vi "qTSP.vi"(0 "System no.":i32=1 min=1 max=4 step=1, 2 "Sensor to query":string[](array[string]), 3 "All sensors?":bool, 4 "Sensor identifier?":bool=TRUE, 5 "error in":errorcluster) -> (14 "Sensor position":dbl[](array[numeric]) format="%.6f", 15 "Sensor to query out":string[](array[string]), 19 "error out":errorcluster)   [LabVIEW 2026]
doc: "Returns sensor position for the specified sensor number.\n\nE-517, E-518: If All sensors? = TRUE, then Sensor identifier? can be FALSE. The input signal channels to be queried with TSP? are the sensor channels of the piezo control electronics, IDs = 1 to 3 (actually available IDs depend on the response to TSC?).\n\nE-761: If All sensors? = TRUE, then Sensor identifier? can be FALSE. \n\nE-709: If All sensors? = TRUE, then Sensor identifier? must be FALSE. Sensors to query comprises all ADC channels of the device: can be the \"genuine\" sensor (sensor integrated in the mechanics, identifier = 1) and the \"general purpose\" analog input (identifier = 2).\n\nE-710: If All sensors? = TRUE, then Sensor identifier? must be TRUE. Command is available in command level 1 only (see CCL.vi, CCL?.vi)\n\nC-413, E-712, E-725, E-727: If All sensors? = TRUE, then Sensor identifier? can be FALSE. Sensors to query comprises all ADC channels of the device: can be a \"genuine\" sensor (sensor integrated in the mechanics) or a \"general purpose\" analog input.\n\nE-753: If All sensors? = TRUE, then Sensor identifier? can be FALSE. Sensors to query comprises all ADC channels of the device: can be the \"genuine\" sensor (capacitive sensor integrated in the mechanics, identifier = 1) and the \"general purpose\" analog input (identifier = 2).\n\nE-754: If All sensors? = TRUE, then Sensor identifier? must be FALSE. Sensors to query comprises all ADC channels of the device: can be the \"genuine\" sensor (capacitive sensor integrated in the mechanics, identifier = 1, or incremental sensor, identifier = 3) and the \"general purpose\" analog input (identifier = 2).\n\nE-755: If All sensors? = TRUE, then Sensor identifier? can be FALSE. Command not available for E-755.101.\n\nMercury_GCS: If All sensors? = TRUE, then Sensor identifier? can be FALSE."
panel:
  # "Returns sensor position for the specified sensor number."
  # "If all sensors: use"
  # "Query"
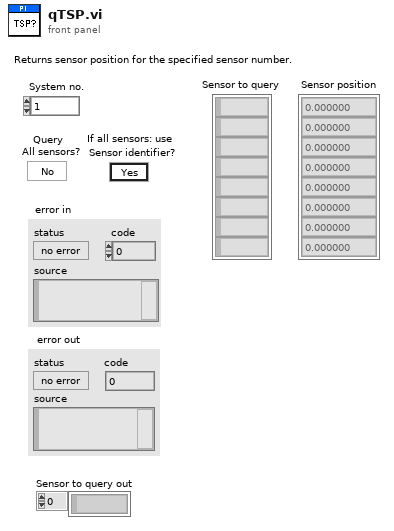
[diagram p1: front panel]
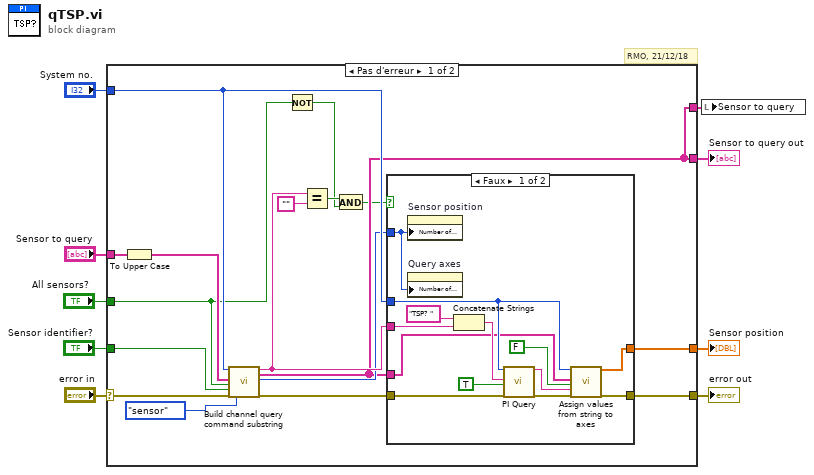
[diagram p0: block diagram]
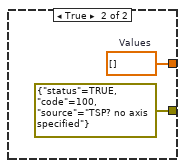
[diagram p2: hidden frame]
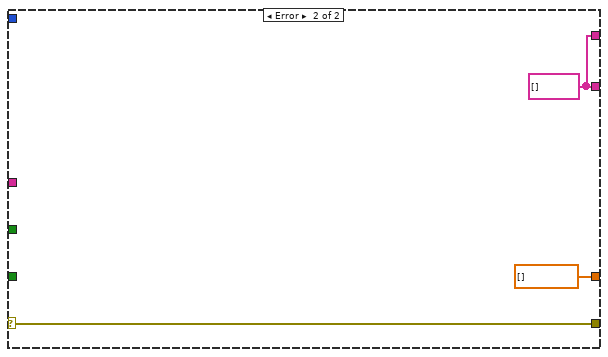
[diagram p3: hidden frame]
diagram:
  # "RMO, 21/12/18"
  n1 = case shown="Pas d'erreur" "error in" {
    selector: "error in" -> [w13 w43]
    tunnel: [w26 dbl[] [] ("Values")] -> w9
    tunnel: "Sensor to query" -> [w25 _]
    tunnel: [w12 w43] -> w7
    tunnel: "Sensor identifier?" -> [w16 _]
    tunnel: "System no." -> [w19 _]
    tunnel: [w11 w42] -> w4
    tunnel: "All sensors?" -> [w17 _]
    tunnel: [w11 w42] -> w1
    frame No Error {
      n2 = To Upper Case(1:w25) -> (0:w18:string[])
      n3 = call "Build channel query command substring.vi"("System no."=w19, "Channels to query in"=w18, "Query\nAll channels?"=w17, "For all channels: use\nChannel identifier?"=w16, "error in"=w13, "Channel type"=enum16{"piezo", "sensor"}."sensor") -> ("Command substring"=w15:string, "Channels to query out"=w11:string[], "Number of rows"=w14:u32, "error out"=w20:errorcluster)  [unwired: 1 in, 9 out]
      n4 = Not(x=w17) -> (.not. x?=w22:bool)
      n5 = Equal?(x=w15, y="" ("x")) -> (x = y?=w23:bool)
      n6 = And(x=w23, y=w22) -> (x .and. y?=w10:bool)
      n7 = case shown="Faux" w10 {
        tunnel: [w36 w40] -> w26
        tunnel: w20 -> [w35 _]
        tunnel: w19 -> [w34 _]
        tunnel: w15 -> [w33 _]
        tunnel: w14 -> [w32 _]
        tunnel: [w30 errorcluster {"status"=TRUE, "code"=100, "source"="TSP? no axis specified"} ("error out")] -> w12
        tunnel: w11 -> [w29 _]
        frame False {
          n8 = property on="Sensor position" class="Tabl (strict)"("Number of Rows"=w32) -> ()  [unwired: 2 in, 2 out]
          n9 = property on="Query axes" class="Tabl (strict)"("Number of Rows"=w32) -> ()  [unwired: 2 in, 2 out]
          n10 = Concatenate Strings("TSP? ", w33) -> (w37:string)
          n11 = call "PI Query.vi"("System no."=w34, "String to send"=w37, "Attach termination char.?"=TRUE ("Attach Linefeed?"), "error in"=w35) -> ("String read"=w27:string, "error out"=w28:errorcluster)  [unwired: 3 in, 11 out]
          n12 = call "Assign values from string to axes.vi"("System no."=w34, "Queried axes"=w29, "All axes queried?"=FALSE, "Input String"=w27, "error in"=w28) -> ("Values"=w36:dbl[], "error out"=w30:errorcluster)  [unwired: 4 in, 9 out]
        }
        frame True {
          w40 = dbl[] []  # Values
        }
      }
    }
    frame Error {
      w42 = string[] [] ("Axes to query out")
    }
  }
  "error out" <- w7
  "Sensor position" <- w9
  "Sensor to query out" <- w1
  n13 = local write "Sensor to query"(w4) -> ()
